vi "ConvertFrontPanel.vi"(7 "Build Directory":path, 8 "error in":errorcluster, 11 "VI Interpreter":refnum<class "VI Interpreter.lvclass">) -> (0 "error out":errorcluster, 3 "VI Interpreter out":refnum<class "VI Interpreter.lvclass">)   [LabVIEW 2014, in "PythonConverter_GUI.lvclass"]
uses:
  PythonConverter_GUI.lvclass
  VI Interpreter/Classes/VI Interpreter/VI Interpreter.lvclass
  PythonConverter_GUI.lvclass/PythonConverter_GUI.ctl
  Parsing/Python Functions.lvlib
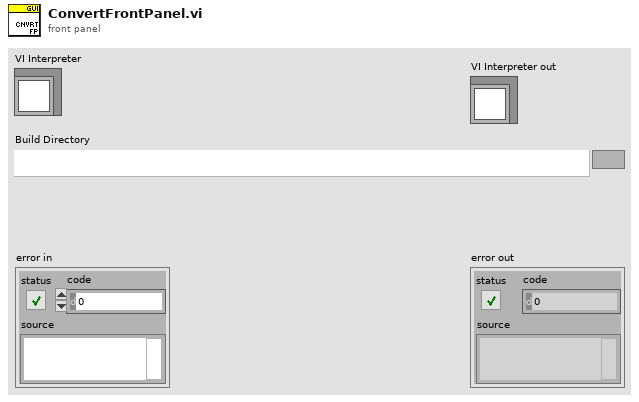
[diagram p1: front panel]
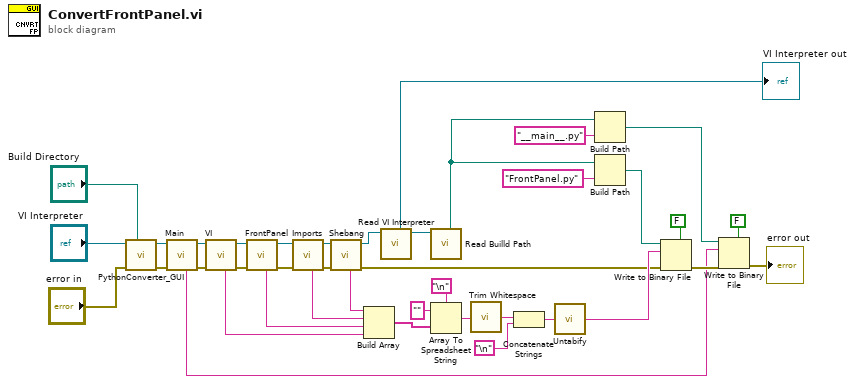
[diagram p0: block diagram]
diagram:
  n1 = call "PythonConverter_GUI.vi"("Build Directory"="Build Directory", "error in"="error in", "VI Interpreter"="VI Interpreter") -> ("error out"=w13:errorcluster, "PythonConverter_GUI out"=w14:refnum<class "PythonConverter_GUI.lvclass">)  [unwired: 5 in]
  n2 = call "Main.vi"("error in"=w13, "PythonConverter_GUI in"=w14) -> ("error out"=w28:errorcluster, "PythonConverter_GUI out"=w31:refnum<class "PythonConverter_GUI.lvclass">, "main"=w6:string)  [unwired: 7 in]
  n3 = call "VI.vi"("error in"=w28, "PythonConverter_GUI in"=w31) -> ("error out"=w27:errorcluster, "PythonConverter_GUI out"=w30:refnum<class "PythonConverter_GUI.lvclass">, "VI"=w35:string)  [unwired: 7 in]
  n4 = call "FrontPanel.vi"("error in"=w27, "PythonConverter_GUI in"=w30) -> ("error out"=w26:errorcluster, "PythonConverter_GUI out"=w29:refnum<class "PythonConverter_GUI.lvclass">, "FrontPanel"=w34:string)  [unwired: 7 in]
  n5 = call "Imports.vi"("error in"=w26, "PythonConverter_GUI in"=w29) -> ("error out"=w32:errorcluster, "PythonConverter_GUI out"=w33:refnum<class "PythonConverter_GUI.lvclass">, "imports"=w38:string)  [unwired: 5 in]
  n6 = call "Shebang.vi"("error in"=w32, "PythonConverter_GUI in"=w33) -> ("error out"=w15:errorcluster, "PythonConverter_GUI out"=w4:refnum<class "PythonConverter_GUI.lvclass">, "shebang"=w39:string)  [unwired: 5 in]
  n7 = Build Array(w39, w38, w34, w35) -> (w25:string[])
  n8 = call "Read VI Interpreter.vi"("PythonConverter_GUI in"=w4) -> ("PythonConverter_GUI out"=w3:refnum<class "PythonConverter_GUI.lvclass">, "VI Interpreter"=→"VI Interpreter out":refnum<class "VI Interpreter.lvclass">)  [unwired: 7 in]
  n9 = call "Read Builld Path.vi"("PythonConverter_GUI in"=w3) -> ("Builld Path"=w12:path)  [unwired: 7 in, 1 out]
  n10 = Array To Spreadsheet String(delimiter (Tab)="\n", array=w25, 3:"" ("format string")) -> (spreadsheet string=w22:string)
  n11 = call <vilib>:"Trim Whitespace.vi"("string"=w22) -> ("trimmed string"=w21:string)  [unwired: 1 in]
  n12 = Concatenate Strings(w21, "\n") -> (w19:string)
  n13 = call "Untabify.vi"("string in"=w19) -> ("string out"=w36:string)  [unwired: 1 in]
  n14 = Build Path(base path=w12, name or relative path="__main__.py") -> (appended path=w7:path)
  n15 = Build Path(base path=w12, name or relative path="FrontPanel.py" ("string")) -> (appended path=w37:path)
  n16 = Write to Binary File(file (use dialog)=w37, data=w36, error in=w15, 5:FALSE ("prepend array or string size? (T)")) -> (error out=w10:errorcluster)  [unwired: 2 in, 2 out]
  n17 = Write to Binary File(file (use dialog)=w7, data=w6, error in=w10, 5:FALSE ("prepend array or string size? (T)")) -> (error out=→"error out":errorcluster)  [unwired: 2 in, 2 out]
